vi "Configure Acquisition.vi"(7 "Enable Continuous Sweep (F: Disable)":bool, 8 "error in (no error)":errorcluster, 9 "Manual Detector Type (0: Positive)":u16(ring) items=["Positive", "RMS", "Negative", "Sample"], 10 "Auto Detector (F: Disable)":bool, 11 "VISA resource name":refnum<visa-resource-name>) -> (0 "error out":errorcluster, 3 "VISA resource name out":refnum<visa-resource-name>)   [LabVIEW 2015, in "Template - Spectrum Analyzer.lvlib"]
doc: "Configures the acquisition properties of the spectrum analyzer."
uses:
  <instrlib>/_Template - Spectrum Analyzer/Template - Spectrum Analyzer.lvlib
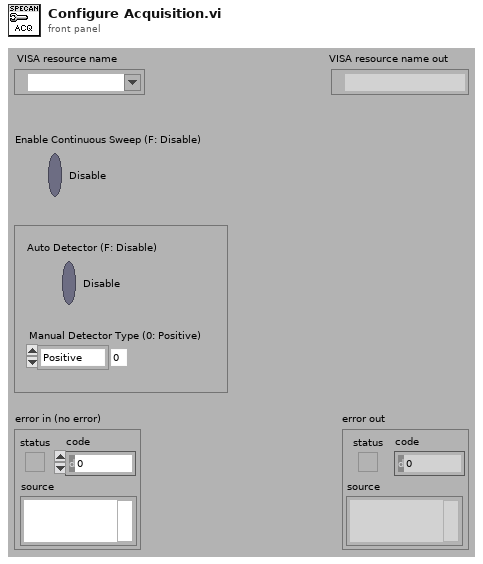
[diagram p1: front panel]
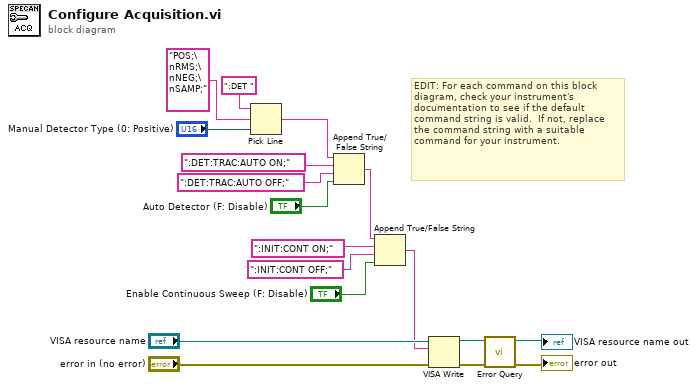
[diagram p0: block diagram]
diagram:
  # "EDIT: For each command on this block diagram, check your instrument's documentation to see if the default command string is valid.  If not, replace the command string with a suitable command for your instrument."
  n1 = Pick Line(string ("")=":DET ", multi-line string="POS;\nRMS;\nNEG;\nSAMP;", line index="Manual Detector Type (0: Positive)") -> (output string=w3:string)
  n2 = Append True/False String(1:"Auto Detector (F: Disable)", 2:":DET:TRAC:AUTO OFF;" ("true string"), 3:":DET:TRAC:AUTO ON;" ("true string"), 4:w3) -> (0:w9:string)
  n3 = Append True/False String(1:"Enable Continuous Sweep (F: Disable)", 2:":INIT:CONT OFF;" ("false string"), 3:":INIT:CONT ON;" ("format string"), 4:w9) -> (0:w11:string)
  n4 = VISA Write(VISA resource name="VISA resource name", write buffer=w11, error in (no error)="error in (no error)") -> (VISA resource name out=w8:refnum<visa-resource-name>, error out=w6:errorcluster)  [unwired: 1 out]
  n5 = call <instrlib>:"Error Query.vi"("error in (no error)"=w6, "VISA resource name"=w8) -> ("error out"=→"error out":errorcluster, "VISA resource name out"=→"VISA resource name out":refnum<visa-resource-name>)  [unwired: 6 in, 2 out]
